vi "LightCtrlHMI.vi"() -> ()   [LabVIEW 2016]
uses:
  <vilib>/Instr/_visa.llb/VISA Configure Serial Port (Serial Instr).vi
  <vilib>/Utility/file.llb/Write Delimited Spreadsheet (DBL).vi
panel:
  in  "Serial Port":refnum<visa-resource-name>="COM5"
  in  "Sampling Time (ms)":dbl=100.0
  in  "Stop":bool
  out "Y":u16(slide) scale=0.0..1023.0
  in  "SP":u16(slide) scale=0.0..1023.0
  out "Plot":cluster{"SP":u16, i32}(graph)
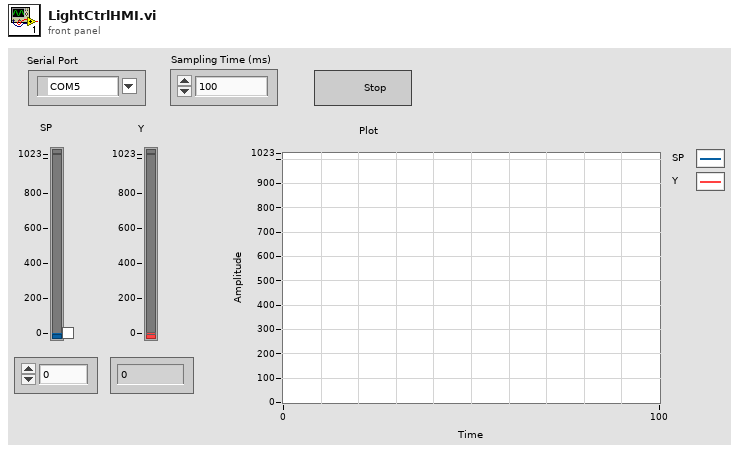
[diagram p1: front panel]
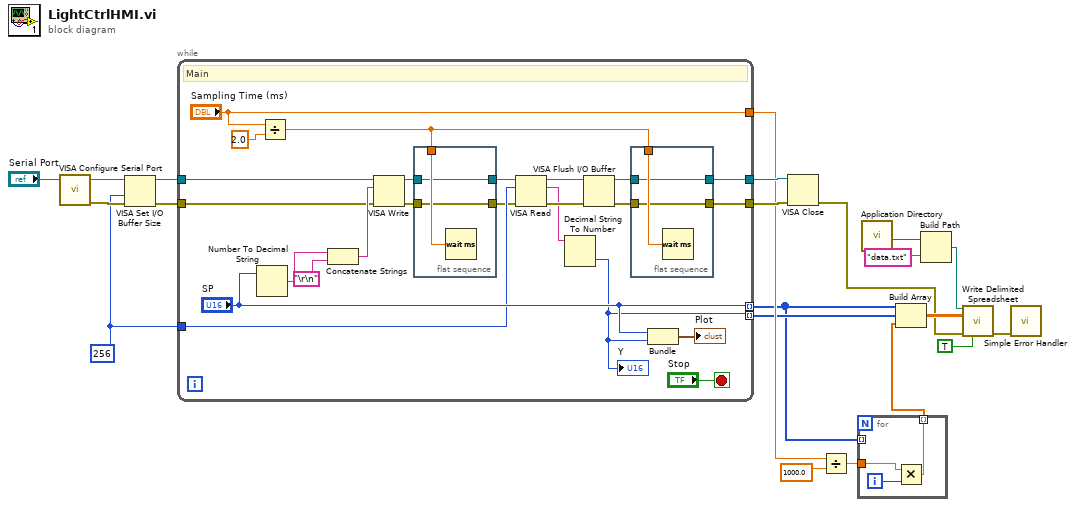
[diagram p0: block diagram]
diagram:
  w1 = u32 256 ("size (4096)")
  n1 = call-poly "VISA Configure Serial Port"("VISA resource name"="Serial Port") -> ("VISA resource name out"=w4:refnum<visa-resource-name>, "error out"=w5:errorcluster)  [unwired: 13 in]
  n2 = VISA Set I/O Buffer Size(VISA resource name=w4, size (4096)=w1, error in (no error)=w5) -> (VISA resource name out=w2:refnum<visa-resource-name>, error out=w3:errorcluster)  [unwired: 1 in]
  n3 = while {
    tunnel: w2 -> [w39]
    tunnel: w3 -> [w40]
    tunnel: ["SP"] -> w13 mode=indexing
    tunnel: [w28] -> w14 mode=indexing
    tunnel: [w27] -> w20
    tunnel: [w26] -> w19
    tunnel: ["Sampling Time (ms)"] -> w16
    tunnel: w1 -> [w23]
    stop <- "Stop" stop-if-true
    # "Main"
    n4 = Number To Decimal String(number="SP") -> (decimal integer string=w41:string)  [unwired: 1 in]
    n5 = Divide(x="Sampling Time (ms)", y=2.0) -> (x/y=w31:dbl)
    n6 = Concatenate Strings(w41, "\r\n") -> (w43:string)
    n7 = VISA Write(VISA resource name=w39, write buffer=w43, error in (no error)=w40) -> (VISA resource name out=w37:refnum<visa-resource-name>, error out=w38:errorcluster)  [unwired: 1 out]
    n8 = flat-sequence {
      tunnel: w31 -> [w51]
      tunnel: [w50] -> w22
      tunnel: w38 -> [w50]
      tunnel: [w49] -> w24
      tunnel: w37 -> [w49]
      frame #0 {
        n9 = Wait (ms)(milliseconds to wait=w51) -> ()  [unwired: 1 out]
      }
    }
    n10 = VISA Read(VISA resource name=w24, byte count=w23, error in (no error)=w22) -> (VISA resource name out=w35:refnum<visa-resource-name>, read buffer=w34:string, error out=w36:errorcluster)  [unwired: 1 out]
    n11 = Decimal String To Number(string=w34) -> (number=w28:i32)  [unwired: 2 in, 1 out]
    "Y" <- w28
    n12 = VISA Flush I/O Buffer(VISA resource name=w35, error in (no error)=w36) -> (VISA resource name out=w32:refnum<visa-resource-name>, error out=w33:errorcluster)  [unwired: 1 in]
    n13 = flat-sequence {
      tunnel: w31 -> [w48]
      tunnel: [w47] -> w27
      tunnel: w33 -> [w47]
      tunnel: [w46] -> w26
      tunnel: w32 -> [w46]
      frame #0 {
        n14 = Wait (ms)(milliseconds to wait=w48) -> ()  [unwired: 1 out]
      }
    }
    n15 = Bundle("SP"="SP", w28) -> (→"Plot":cluster{"SP":u16, i32})  [unwired: 1 in]
  }
  n16 = VISA Close(VISA resource name=w19, error in (no error)=w20) -> (error out=w7:errorcluster)
  n17 = Divide(x=w16, y=1000.0) -> (x/y=w18:dbl)
  n18 = for {
    tunnel: w13 -> [_] mode=indexing
    tunnel: w18 -> [w53]
    tunnel: [w52] -> w15 mode=indexing
    i -> [w54]
    n19 = Multiply(x=w53, y=w54) -> (x*y=w52:dbl)
  }
  n20 = call <vilib>:"Application Directory.vi"() -> ("Application Directory"=w10:path)
  n21 = Build Array(w13, w14, w15) -> (w12:dbl[][])
  n22 = Build Path(base path=w10, name or relative path="data.txt") -> (appended path=w8:path)
  n23 = call-poly <vilib>:"Write Delimited Spreadsheet.vi"("file path (dialog if empty)"=w8, "2D data"=w12, "error in (no error)"=w7, "transpose? (no:F)"=TRUE) -> ("error out"=w6:errorcluster)  [unwired: 10 in, 1 out]
  n24 = call <vilib>:"Simple Error Handler.vi"("error in (no error)"=w6) -> ()  [unwired: 4 in, 5 out]
